vi "LoadCalibrationFile.vi"(8 "error in (no error)":errorcluster, 11 "Path":path) -> (0 "error out":errorcluster, 3 "CalibrationState":T1)   [LabVIEW 2012]
panel:
  # "CalibrationDone"
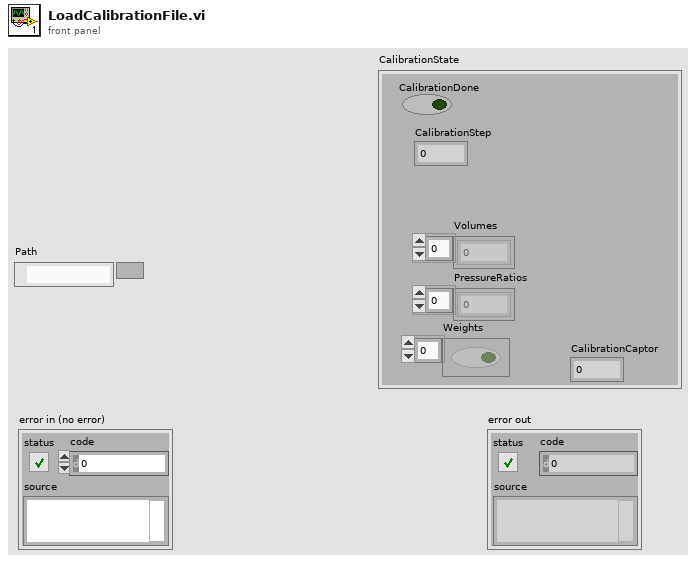
[diagram p1: front panel]
types:
  T1 = cluster{bool, "CalibrationStep":u32, "Volumes":dbl[], "PressureRatios":dbl[], "Weights":bool[], "CalibrationCaptor":u32}
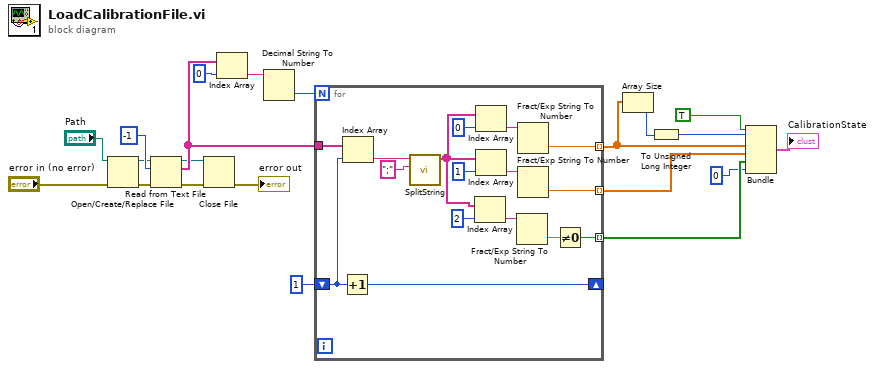
[diagram p0: block diagram]
diagram:
  n1 = Open/Create/Replace File(file path (use dialog)="Path", error in="error in (no error)") -> (refnum out=w16:refnum<file>, error out=w17:errorcluster)  [unwired: 4 in, 1 out]
  n2 = Read from Text File(file (use dialog)=w16, count=-1, error in=w17) -> (refnum out=w7:refnum<file>, text=w11:string[], error out=w6:errorcluster)  [unwired: 1 in, 1 out]
  n3 = Close File(refnum=w7, error in=w6) -> (error out=→"error out":errorcluster)  [unwired: 1 out]
  n4 = Index Array(array=w11, index=0) -> (element=w12:string)
  n5 = Decimal String To Number(string=w12) -> (number=w15:i32)  [unwired: 2 in, 1 out]
  n6 = for {
    N: w15 -> [_]
    shift-right: [w37] -> _
    shift-left: 1 -> [w33]
    tunnel: w11 -> [w36]
    tunnel: [w28] -> w5 mode=indexing
    tunnel: [w27] -> w10 mode=indexing
    tunnel: [w22] -> w2 mode=indexing
    n7 = Increment(x=w33) -> (x+1=w37:i32)
    n8 = Index Array(array=w36, index=w33) -> (element=w35:string)
    n9 = call "SplitString.vi"("Separator"=";", "String[in]"=w35) -> ("Slices"=w24:string[])  [unwired: 9 in]
    n10 = Index Array(array=w24, index=2) -> (element=w26:string)
    n11 = Index Array(array=w24, index=0) -> (element=w30:string)
    n12 = Index Array(array=w24, index=1) -> (element=w29:string)
    n13 = Fract/Exp String To Number(string=w26) -> (number=w23:dbl)  [unwired: 3 in, 1 out]
    n14 = Fract/Exp String To Number(string=w30) -> (number=w28:dbl)  [unwired: 3 in, 1 out]
    n15 = Fract/Exp String To Number(string=w29) -> (number=w27:dbl)  [unwired: 3 in, 1 out]
    n16 = Not Equal To 0?(x=w23) -> (x != 0?=w22:bool)
  }
  n17 = Array Size(array=w5) -> (size(s)=w3:i32)
  n18 = To Unsigned Long Integer(number=w3) -> (unsigned 32bit integer=w4:u32)
  n19 = Bundle(TRUE, w4, w5, w10, w2, 0) -> (→"CalibrationState":cluster{bool, u32, dbl[], dbl[], bool[], i32})  [unwired: 1 in]
